vi "Lake Shore 336 Configure Heater Output Control Parameters and Acquire Single Reading.vi"(0 "VISA resource name":refnum<visa-resource-name>) -> ()   [LabVIEW 2020]
doc: "This VI was designed to demonstrate typical usage of sub VIs containing the more common 336 functions. The VI Initializes the instrument, allows the user to determine if heater output control parameters and setpoint values are sent, takes a single sensor reading, and then closes the instrument."
uses:
  Public/Data/Sensor Data (Single Reading).vi
  Lake Shore 336.lvlib
panel:
  in  "Output's Control Loop (1:1)":u16(ring)=1 items=["1"=1, "2"=2]
  in  "Input (0:A)":u16(ring) items=["A", "B", "C", "D"]
  in  "Data Source (0:Kelvin)":u16(ring) items=["Kelvin", "Celsius", "Sensor Units"]
  out "Sensor Data":dbl format="%.4f"
  in  "Setpoint (0.00000)":dbl format="%.5f"
  in  "Range (0:Off)":u16(ring) items=["Off", "Low (On)", "Medium", "High"]
  in  "Manual Output (0.00 %)":dbl format="%.2f"
  in  "Rate (D) (0.0 %)":dbl format="%.1f"
  in  "Reset (I) (20.0)":dbl=20.0 format="%.1f"
  in  "Gain (P) (50.0)":dbl=50.0 format="%.1f"
  in  "Heater Resistance (1:25 Ohms)":u16(ring)=1 items=["25 Ohms"=1, "50 Ohms"=2]
  in  "Max User Current (2.000)":dbl=2.0 format="%.3f"
  in  "Heater Out Display (1:Current)":u16(ring)=1 items=["Current"=1, "Power"=2]
  in  "Max Current (0:User Specified)":u16(ring) items=["User Specified", "0.707 A", "1.0 A", "1.141 A", "2.0 A"]
  in  "Mode (0:Off)":u16(ring) items=["Off", "Closed Loop PID", "Zone", "Open Loop"]
  in  "Power Up Enable (F: Off)":bool
  in  "Input (0:None)":u16(ring) items=["None", "A", "B", "C", "D"]
  in  "Serial Configuration":T1={"Baud Rate"=57600, "Parity"=1, "Data Bits"=7, "Stop Bits"=10, "Flow Control"=0} {"Flow Control" items=["None", "XON/XOFF", "RTS/CTS", "XON/XOFF & RTS/CTS", "DTR/DSR", "XON/XOFF & DTR/DSR"]; "Stop Bits" items=["1.0"=10, "1.5"=15, "2.0"=20]; "Data Bits" items=["7"=7, "8"=8]; "Parity" items=["None", "Odd", "Even", "Mark", "Space"]; "Baud Rate" items=["300"=300, "600"=600, "1200"=1200, "2400"=2400, "4800"=4800, "9600"=9600, "19200"=19200, "38400"=38400, "57600"=57600]}
  in  "Enable Setpoint (F:Off)":bool
  in  "Configure Control Parameters (1: Don't Configure)":u16(ring) items=["Configure", "Don't Configure"]
  # "(c) 2009 Lake Shore Cryotronics Inc.  ALL RIGHTS RESERVED."
  # "Sensor Data"
  # "Control Parameters"
  # "Setpoint"
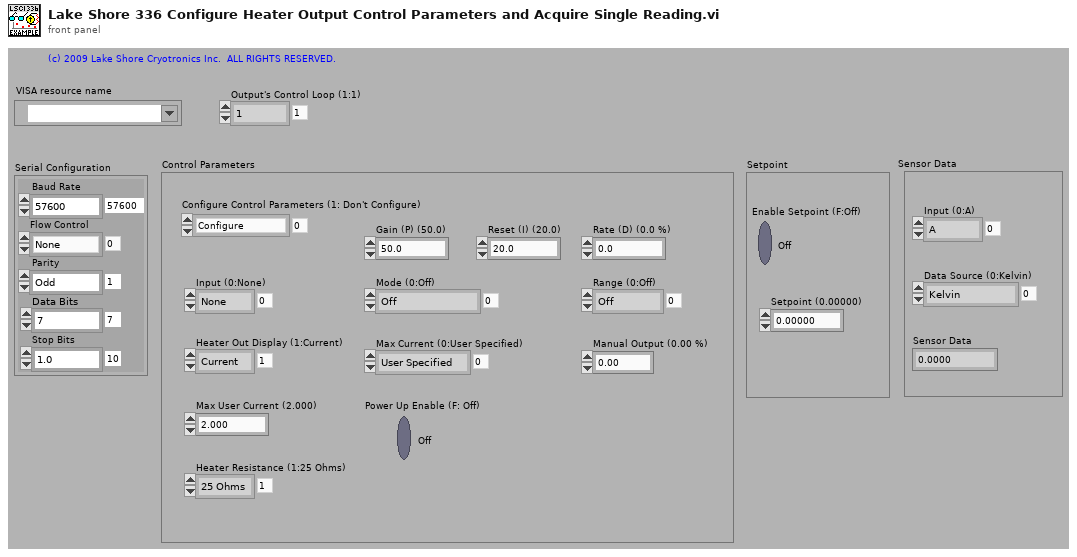
[diagram p1: front panel]
types:
  T1 = cluster{"Baud Rate":u32, "Parity":u16, "Data Bits":u16, "Stop Bits":u16, "Flow Control":u16}
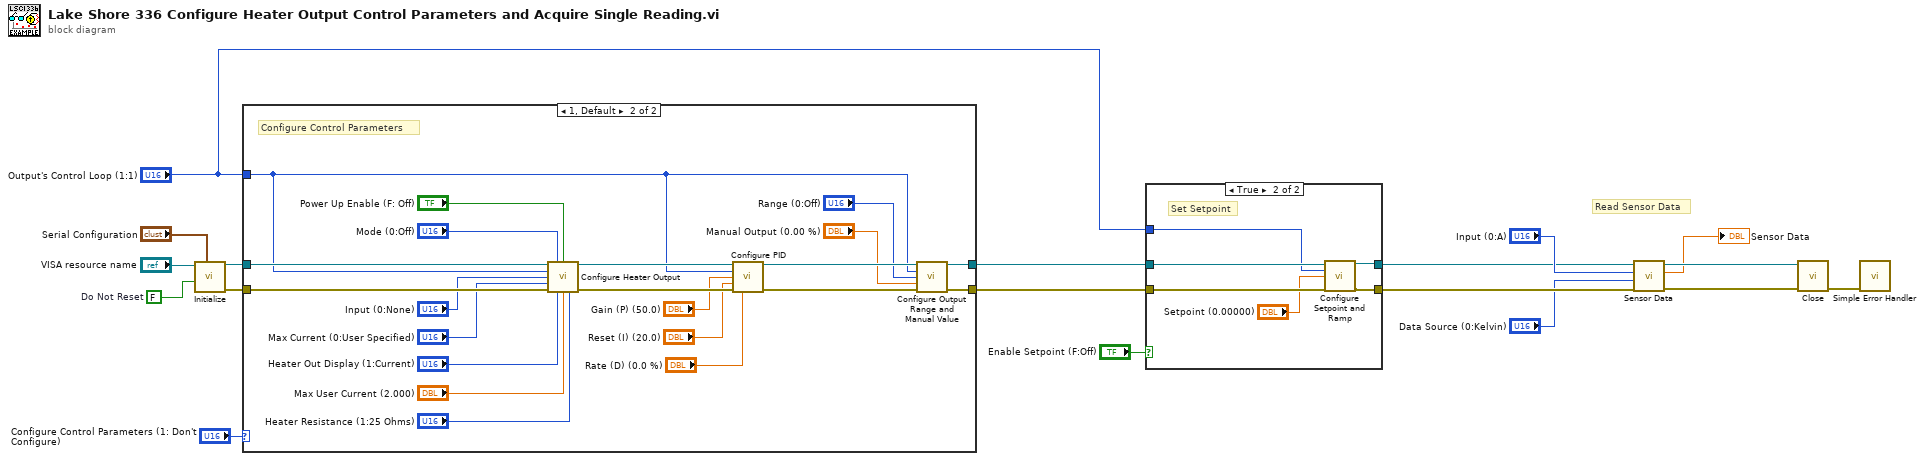
[diagram p0: block diagram]
diagram:
  w10 = FALSE  # Do Not Reset
  # "Read Sensor Data"
  n1 = call "Initialize.vi"("Serial Configuration"="Serial Configuration", "Reset (True)"=w10, "VISA resource name"="VISA resource name") -> ("error out"=w17:errorcluster, "VISA resource name out"=w18:refnum<visa-resource-name>)  [unwired: 7 in]
  n2 = case shown="1, Default" "Configure Control Parameters (1: Don't Configure)" {
    tunnel: "Output's Control Loop (1:1)" -> [_ w26]
    tunnel: w18 -> [w20 w41]
    tunnel: w17 -> [w19 w40]
    tunnel: [w19 w35] -> w11
    tunnel: [w20 w34] -> w12
    frame 0 {
      # "Do Not Configure Control Parameters"
    }
    frame 1, Default {
      # "Configure Control Parameters"
      n3 = call "Configure Heater Output.vi"("VISA resource name"=w41, "Mode (0:Off)"="Mode (0:Off)", "Power Up Enable (F: Off)"="Power Up Enable (F: Off)", "Heater Output (1:1)"=w26, "Input (0:None)"="Input (0:None)", "Max Current (0:User Specified)"="Max Current (0:User Specified)", "error in (no error)"=w40, "Heater Out Display (1:Current)"="Heater Out Display (1:Current)", "Max User Current (2.000)"="Max User Current (2.000)", "Heater Resistance (1:25 Ohms)"="Heater Resistance (1:25 Ohms)") -> ("VISA resource name out"=w38:refnum<visa-resource-name>, "error out"=w39:errorcluster)  [unwired: 4 in]
      n4 = call "Configure PID.vi"("VISA resource name"=w38, "Output's Control Loop (1:1)"=w26, "Gain (P) (50.0)"="Gain (P) (50.0)", "Reset (I) (20.0)"="Reset (I) (20.0)", "error in (no error)"=w39, "Rate (D) (0.0 %)"="Rate (D) (0.0 %)") -> ("VISA resource name out"=w37:refnum<visa-resource-name>, "error out"=w36:errorcluster)  [unwired: 8 in]
      n5 = call "Configure Output Range and Manual Value.vi"("VISA resource name"=w37, "Output (1:1)"=w26, "Range (0:Off)"="Range (0:Off)", "Manual Output (0.00 %)"="Manual Output (0.00 %)", "error in (no error)"=w36) -> ("VISA resource name out"=w34:refnum<visa-resource-name>, "error out"=w35:errorcluster)  [unwired: 9 in]
    }
  }
  n6 = case shown="True" "Enable Setpoint (F:Off)" {
    tunnel: "Output's Control Loop (1:1)" -> [_ w47]
    tunnel: w12 -> [w43 w48]
    tunnel: w11 -> [w42 w49]
    tunnel: [w42 w44] -> w6
    tunnel: [w43 w45] -> w7
    frame False {
      # "Do Not Set Setpoint"
    }
    frame True {
      # "Set Setpoint"
      n7 = call "Configure Setpoint and Ramp.vi"("VISA resource name"=w48, "Output's Control Loop (1:1)"=w47, "Setpoint (0.00000)"="Setpoint (0.00000)", "error in (no error)"=w49) -> ("VISA resource name out"=w45:refnum<visa-resource-name>, "error out"=w44:errorcluster)  [unwired: 10 in]
    }
  }
  n8 = call-poly "Sensor Data.vi"("error in (no error)"=w6, "Data Source (0:Kelvin)"="Data Source (0:Kelvin)", "Input (0:A)"="Input (0:A)", "VISA resource name"=w7) -> ("error out"=w3:errorcluster, "Sensor Data"=→"Sensor Data":dbl, "VISA resource name out"=w4:refnum<visa-resource-name>)  [unwired: 5 in]
  n9 = call "Close.vi"("error in (no error)"=w3, "VISA resource name"=w4) -> ("error out"=w13:errorcluster)  [unwired: 9 in]
  n10 = call <vilib>:"Simple Error Handler.vi"("error in (no error)"=w13) -> ()  [unwired: 4 in, 5 out]
